vi "Bind Controls to SmartDashboard.vi"(6 "Update Time (ms)":i32=100, 8 "Client Name":string="Dashboard", 9 "Path Prefix":string="SmartDashboard", 10 "Bound Control Refs":refnum<vi>[](array[refnum]), 11 "Server IP Address":string="localhost") -> ()   [LabVIEW 2020]
doc: "Place this VI in the Dashboard or other client applications so that it can run in parallel with the other tasks. Provide the robot IP address so that it can know where to find the server. This starts the NT Client automatically.\n\nCombine the path prefix and control name to construct entry names. Bind controls and indicators to a SmartDashboard or Network Table entry with the matching name. Controls and Indicators will be updated each time the table entriy of the same name changes. Table entries will be updated each time the control changes value."
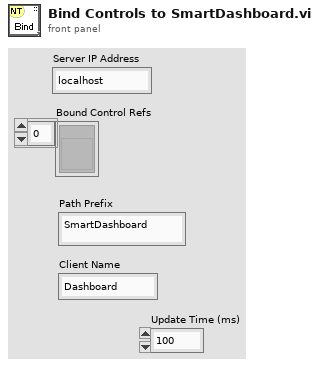
[diagram p1: front panel]
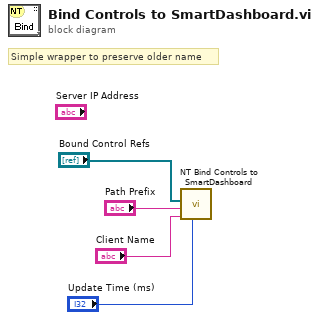
[diagram p0: block diagram]
diagram:
  # "Simple wrapper to preserve older name"
  n1 = call <vilib>:"NT Bind Controls to SmartDashboard.vi"("Update Time (ms)"="Update Time (ms)", "Client Name"="Client Name", "Path Prefix"="Path Prefix", "Bound Control Refs"="Bound Control Refs") -> ()  [unwired: 8 in]
